vi "Get Active Item.vi"(8 "error in (no error)":errorcluster, 11 "Chronological List In":refnum<class "Chronological List.lvclass">) -> (0 "error out":errorcluster, 2 "Debug Data":T1, 3 "Chronological List Out":refnum<class "Chronological List.lvclass">)   [LabVIEW 2020, in "Chronological List.lvclass"]
uses:
  Chronological List.lvclass
  Debugger/TypeDefs/Debug Data.ctl
  Chronological List.lvclass/Chronological List.ctl
  Debugger/Debugger.lvclass
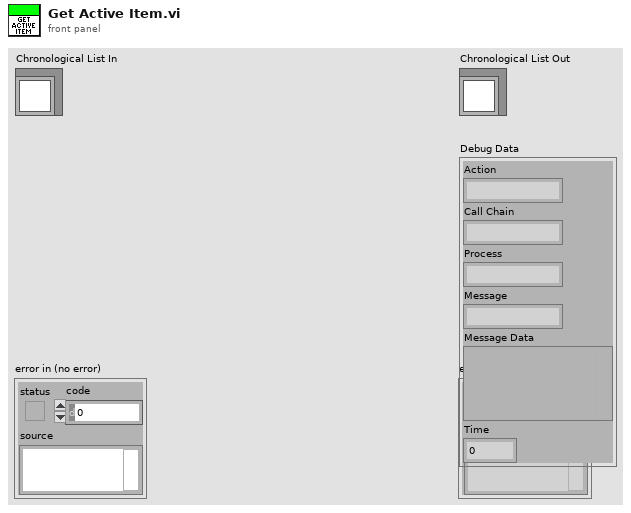
[diagram p1: front panel]
types:
  T1 = typedef "Debugger.lvclass/Debug Data.ctl" = cluster{"Action":string, "Call Chain":string, "Process":string, "Message":string, "Message Data":variant, "Time":u32}
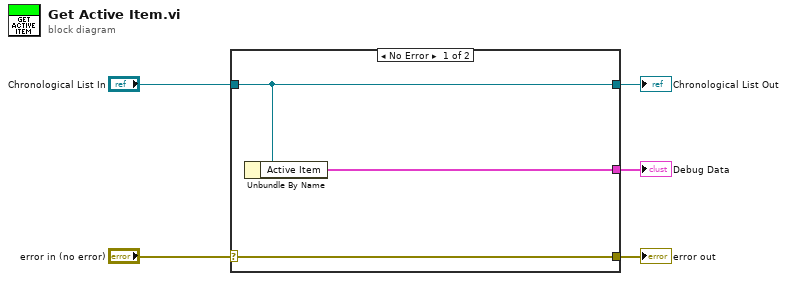
[diagram p0: block diagram]
diagram:
  n1 = case shown="No Error" "error in (no error)" {
    selector: "error in (no error)" -> [w8 w9]
    tunnel: [w8 w9] -> w4
    tunnel: [w7 w10] -> w2
    tunnel: "Chronological List In" -> [w7 w10]
    tunnel: [w6 _] -> w1
    frame No Error {
      n2 = Unbundle By Name(w7) -> ("Active Item"=w6:T1)
    }
    frame Error {
    }
  }
  "error out" <- w4
  "Chronological List Out" <- w2
  "Debug Data" <- w1
